vi "Read MUS deltaTime.vi"(11 "MUS_Data_in":u8[](array[numeric])) -> (2 "delay_tick":u32, 3 "Data_Remaining":u8[](array[numeric]))   [LabVIEW 8.6]
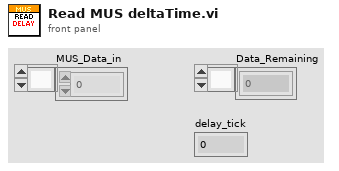
[diagram p1: front panel]
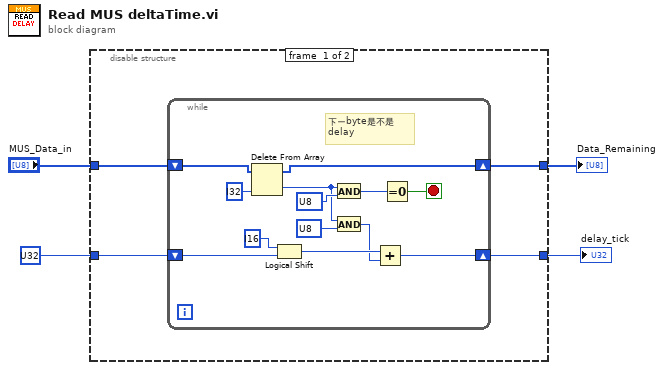
[diagram p0: block diagram]
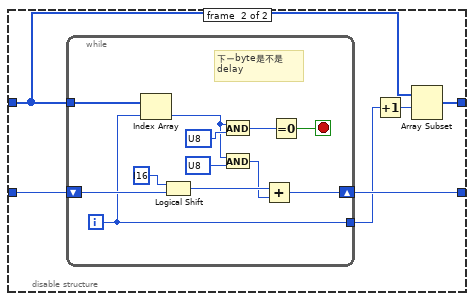
[diagram p2: hidden frame]
diagram:
  n1 = disable-structure shown="Enabled" {
    disable-tunnel: [w8 w26] -> w4
    disable-tunnel: u32 ? ("delay") -> [w7 w27]
    disable-tunnel: [w6 w22] -> w2
    disable-tunnel: "MUS_Data_in" -> [w5 w23]
    frame #0 {
      n2 = while {
        shift-right: [w19] -> w6
        shift-left: w5 -> [w20]
        shift-right: [w15] -> w8
        shift-left: w7 -> [w18]
        stop <- w9 stop-if-true
        # "下ㄧbyte是不是\ndelay"
        n3 = Delete From Array(array=w20, index=i32 ?) -> (deleted portion=w11:u8, array with subset deleted=w19:u8[])  [unwired: 1 in]
        n4 = Logical Shift(y=i16 ?, x=w18) -> (x << y=w16:u32)
        n5 = And(x=w11, y=u8 ?) -> (x .and. y?=w10:u8)
        n6 = And(x=w11, y=u8 ?) -> (x .and. y?=w12:u8)
        n7 = Add(x=w16, y=w12) -> (x+y=w15:u32)
        n8 = Equal To 0?(x=w10) -> (x = 0?=w9:bool)
      }
    }
    frame #1 {
      n9 = while {
        shift-right: [w35] -> w26
        shift-left: w27 -> [w38]
        tunnel: w23 -> [w39]
        tunnel: [w28] -> w24
        i -> [w28]
        stop <- w29 stop-if-true
        # "下ㄧbyte是不是\ndelay"
        n10 = Index Array(array=w39, index=w28) -> (element=w31:u8)
        n11 = Logical Shift(y=i16 ?, x=w38) -> (x << y=w36:u32)
        n12 = And(x=w31, y=u8 ?) -> (x .and. y?=w30:u8)
        n13 = And(x=w31, y=u8 ?) -> (x .and. y?=w32:u8)
        n14 = Add(x=w36, y=w32) -> (x+y=w35:u32)
        n15 = Equal To 0?(x=w30) -> (x = 0?=w29:bool)
      }
      n16 = Increment(x=w24) -> (x+1=w25:i32)
      n17 = Array Subset(array=w23, index=w25) -> (w22:u8[])  [unwired: 1 in]
    }
  }
  "delay_tick" <- w4
  "Data_Remaining" <- w2
